vi "PathSup2Lines_Array.vi"(9 "Z":dbl, 10 "HighPower":dbl, 11 "PathSupIn":T2[](array[typedef])) -> (2 "Colors":u32[](array[numeric]), 3 "Lines":cluster{"P0":T1, "P1":T1}[](array[cluster]))   [LabVIEW 2014]
uses:
  TypeDefs/PathSupreme.ctl
  PSup2SCAN/Sub/VelocityProfile.ctl
  PSup2SCAN/Sub/PathCut.ctl
  PSup2SCAN/Sub/Segment.ctl
  TypeDefs/Point3D.ctl
  ColorMaps.ctl
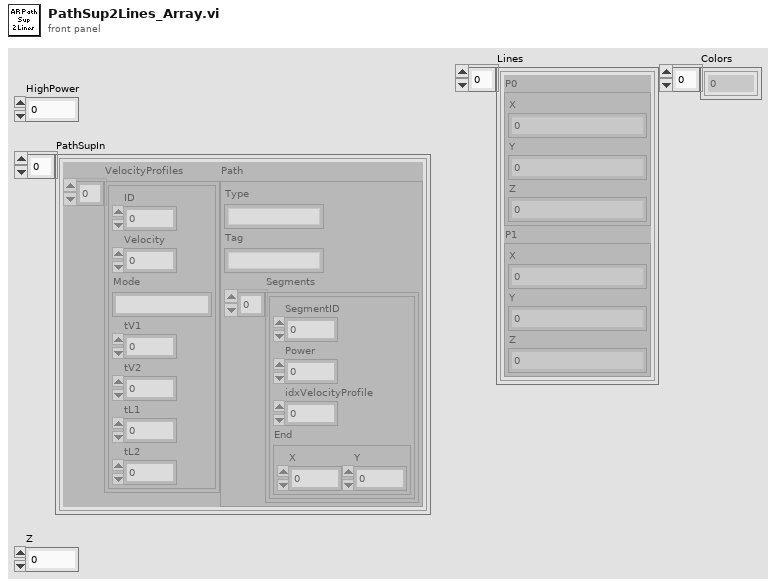
[diagram p1: front panel]
types:
  T1 = typedef "Point3D.ctl" = cluster{"X":sgl, "Y":sgl, "Z":sgl}
  T2 = typedef "PathSupreme.ctl" = cluster{"VelocityProfiles":T3[], "Path":T4}
  T3 = typedef "VelocityProfile.ctl" = cluster{"ID":u32, "Velocity":dbl, "Mode":string, "tV1":u32, "tV2":u32, "tL1":u32, "tL2":u32}
  T4 = typedef "PathCut.ctl" = cluster{"Type":string, "Tag":string, "Segments":T5[]}
  T5 = typedef "Segment.ctl" = cluster{"SegmentID":u16, "Power":sgl, "idxVelocityProfile":u16, "End":cluster{"X":sgl, "Y":sgl}}
  T6 = typedef "ColorMaps.ctl" = u16
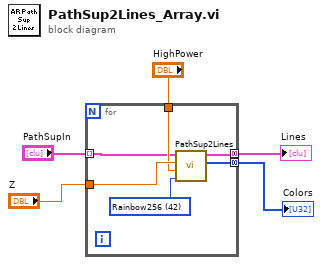
[diagram p0: block diagram]
diagram:
  n1 = for {
    tunnel: "PathSupIn" -> [w6] mode=indexing
    tunnel: "Z" -> [w10]
    tunnel: "HighPower" -> [w9]
    tunnel: [w8] -> w2 mode=concatenating
    tunnel: [w7] -> w1 mode=concatenating
    w11 = T6 42 items=["Bathymetry9", "BlackBody", "Blue", "BlueBlackRed", "BlueGreenOrange", "BlueHot", "BlueHot256", "BlueRedGreen", "BlueRedGreen256", "BrownViolet", "Classification", "ColdWarm", "Copper", "Cyan", "CyanMagenta", "Cycles", "dBZ14", "dBZ21", "EOSOrangeBlue11", "EOSSpectral11", "Fiddle", "Geo", "Geo32", "Gold", "Grays", "Grays16", "Grays256", "Green", "GreenMagenta16", "LandAndSea", "LandAndSea8", "Magenta", "Mocha", "Mud", "Pastels", "PastelsMap", "PastelsMap20", "PlanetEarth", "PlanetEarth256", "Rainbow", "Rainbow4Cycles", "Rainbow16", "Rainbow256", "RainbowCycle", "Red", "RedWhiteBlue", "RedWhiteBlue256", "RedWhiteGreen", "Relief", "Relief19", "SeaLandAndFire", "Spectrum", "SpectrumBlack", "Terrain", "Terrain256", "VioletOrangeYellow", "Web216", "Yellow", "YellowHot", "YellowHot256"] ("ColorMap")
    n2 = call "PathSup2Lines.vi"("ColorMap"=w11, "HighPower"=w9, "Z"=w10, "PathSupreme"=w6) -> ("Colors"=w7:u32[], "Lines"=w8:cluster{"P0":T1, "P1":T1}[])  [unwired: 6 in]
  }
  "Lines" <- w2
  "Colors" <- w1
